vi "资讯打标签-打印函数.vi"(5 "条码类型":bool, 6 "错误输入（无错误）":errorcluster caption="print error in", 7 "label num":i32, 8 "print path local":bool, 9 "PRINT":refnum<k24>, 10 "SN":refnum<k24>, 11 "SN输入":string="000019120-SD-R/Z00A2R1553S") -> (3 "printPath":string, 4 "print error":errorcluster caption="print error out")   [LabVIEW 2011]
uses:
  D:/gitProjects/HPTS_VNA/Data/ClassLibraryMisWebservice.dll
  Data/ClassLibraryMisWebservice.dll
  subVI/logrecord/logrecordstring.vi
panel:
  out "Temp":string
  out "strPrintContent":string
  out "PrintSFCFSNLabel":string="OK"
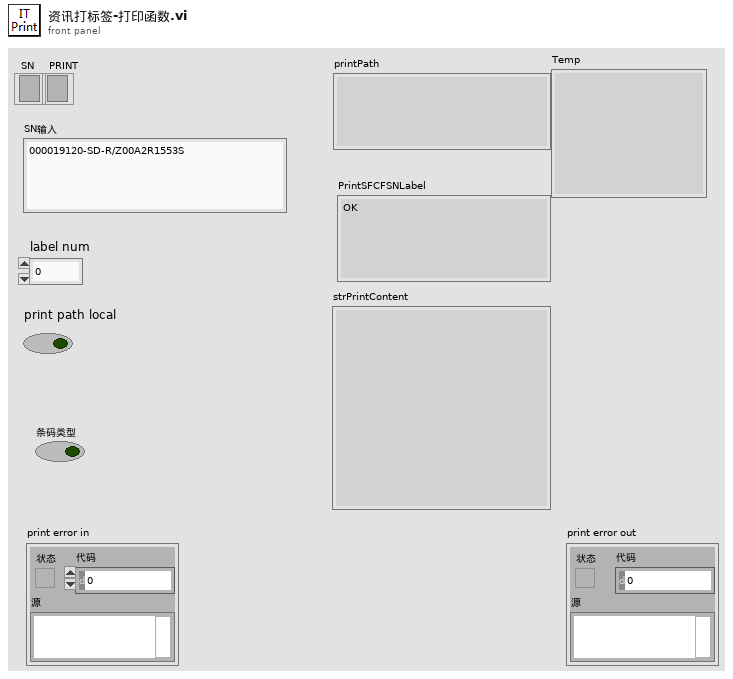
[diagram p1: front panel]
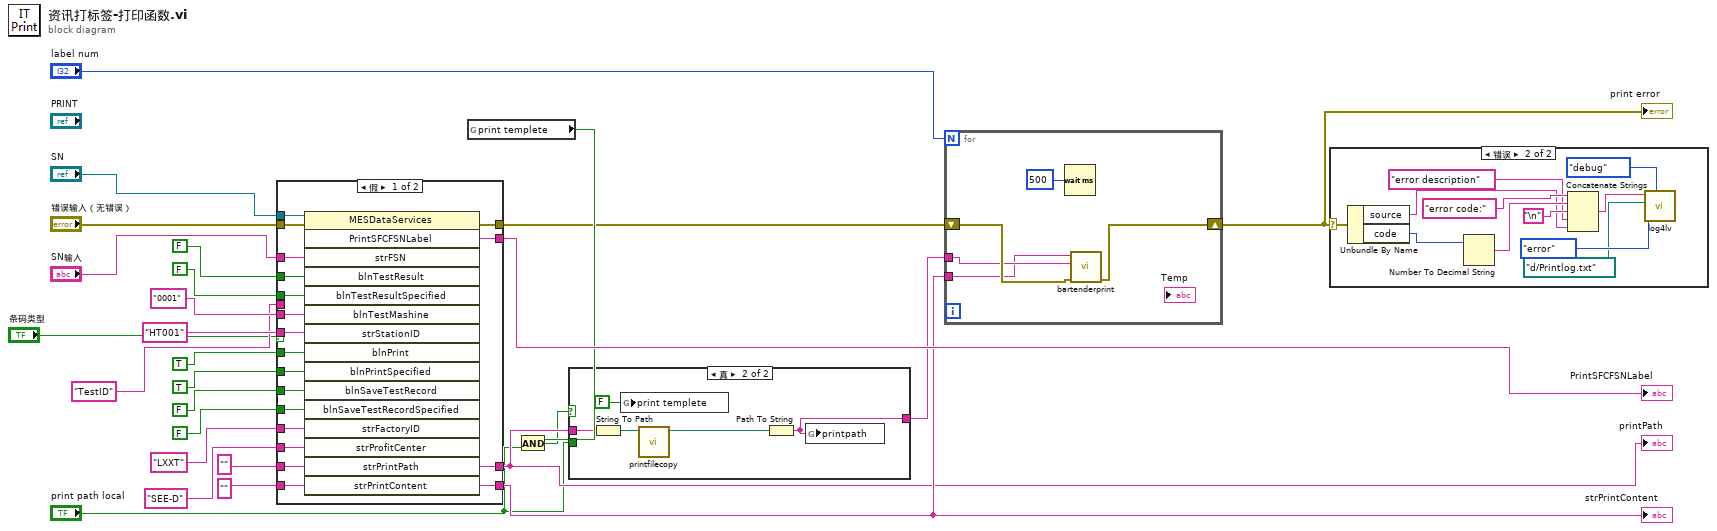
[diagram p0: block diagram]
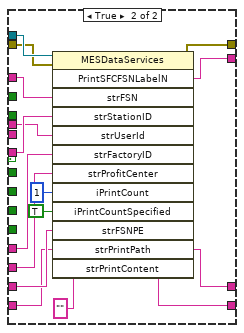
[diagram p2: hidden frame]
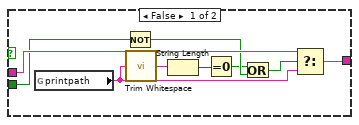
[diagram p4: hidden frame]
diagram:
  n1 = case shown="假" "条码类型" {
    tunnel: FALSE ("blnTestResult") -> [w46 _]
    tunnel: FALSE ("blnTestResultSpecified") -> [w45 _]
    tunnel: "0001" ("blnTestMashine") -> [w44 _]
    tunnel: "HT001" ("strStationID") -> [w43 w57]
    tunnel: TRUE ("blnPrint") -> [w42 _]
    tunnel: TRUE ("blnPrintSpecified") -> [w41 _]
    tunnel: FALSE ("blnSaveTestRecord") -> [w40 _]
    tunnel: FALSE ("blnSaveTestRecordSpecified") -> [w39 _]
    tunnel: "LXXT" ("strFactoryID") -> [w38 w55]
    tunnel: "SEE-D" ("strProfitCenter") -> [w37 w54]
    tunnel: "" ("printPath") -> [w36 w51]
    tunnel: [w35 w58] -> w16
    tunnel: "SN输入" -> [w34 w59]
    tunnel: "" ("strPrintContent") -> [w33 w50]
    tunnel: [w32 w47] -> w13
    tunnel: "SN" -> [w31 w62]
    tunnel: [w30 w48] -> w11
    tunnel: [w29 w60] -> w5
    tunnel: "错误输入（无错误）" -> [w28 w61]
    tunnel: "TestID" -> [_ w56]
    frame False {
      n2 = invoke class="MESDataServices" method="PrintSFCFSNLabel"(reference=w31, error in=w28, "strFSN"=w34, "blnTestResult"=w46, "blnTestResultSpecified"=w45, "blnTestMashine"=w44, "strStationID"=w43, "blnPrint"=w42, "blnPrintSpecified"=w41, "blnSaveTestRecord"=w40, "blnSaveTestRecordSpecified"=w39, "strFactoryID"=w38, "strProfitCenter"=w37, "strPrintPath"=w36, "strPrintContent"=w33) -> (error out=w29:errorcluster, "PrintSFCFSNLabel"=w35:string, "strPrintPath"=w30:string, "strPrintContent"=w32:string)  [unwired: 1 in, 12 out]
    }
    frame True {
      n3 = invoke class="MESDataServices" method="PrintSFCFSNLabelN"(reference=w62, error in=w61, "strFSN"=w59, "strStationID"=w57, "strUserId"=w56, "strFactoryID"=w55, "strProfitCenter"=w54, "iPrintCount"=1, "iPrintCountSpecified"=TRUE, "strFSNPE"=w51, "strPrintPath"=w50, "strPrintContent"="") -> (error out=w60:errorcluster, "PrintSFCFSNLabelN"=w58:string, "strPrintPath"=w48:string, "strPrintContent"=w47:string)  [unwired: 1 in, 9 out]
    }
  }
  "printPath" <- w11
  "PrintSFCFSNLabel" <- w16
  "strPrintContent" <- w13
  n4 = global read "全局.vi" "print templete"() -> (w9:bool)
  n5 = And(x=w9, y="print path local") -> (x .and. y?=w8:bool)
  n6 = case shown="真" w8 {
    tunnel: w11 -> [w69 w76]
    tunnel: [w67 w72] -> w10
    tunnel: "print path local" -> [w66 _]
    frame False {
      n7 = global read "全局.vi" "printpath"() -> (w68:string)
      n8 = Not(x=w66) -> (.not. x?=w65:bool)
      n9 = call <vilib>:"Trim Whitespace.vi"("string"=w68) -> ("trimmed string"=w71:string)  [unwired: 1 in]
      n10 = String Length(string=w71) -> (length=w70:i32)
      n11 = Equal To 0?(x=w70) -> (x = 0?=w64:bool)
      n12 = Or(x=w64, y=w65) -> (x .or. y?=w63:bool)
      n13 = Select(t=w69, s=w63, f=w68) -> (s? t:f=w67:string)
    }
    frame True {
      n14 = String To Path(string=w76) -> (path=w75:path)
      n15 = global write "全局.vi" "print templete"(FALSE ("print templete")) -> ()
      n16 = call "printfilecopy.vi"("源路径"=w75) -> ("new path"=w74:path)  [unwired: 9 in, 1 out]
      n17 = Path To String(path=w74) -> (string=w72:string)
      n18 = global write "全局.vi" "printpath"(w72) -> ()
    }
  }
  n19 = for {
    N: "label num" -> [_]
    tunnel: w13 -> [w77]
    tunnel: w10 -> [w78]
    shift-right: [w80] -> w3
    shift-left: w5 -> [w79]
    n20 = Wait (ms)(milliseconds to wait=u32 500 ("等待时间（毫秒）")) -> ()  [unwired: 1 out]
    n21 = call "bartenderprint.vi"("错误输入"=w79, "Bartender File Path"=w78, "PrintString"=w77) -> ("错误输出"=w80:errorcluster)  [unwired: 8 in]
  }
  "print error" <- w3
  n22 = case shown="错误" w3 {
    selector: w3 -> [_ w92]
    frame No Error {
    }
    frame Error {
      n23 = Unbundle By Name(w92) -> ("source"=w87:string, "code"=w86:i32)
      n24 = Number To Decimal String(number=w86) -> (decimal integer string=w90:string)  [unwired: 1 in]
      n25 = Concatenate Strings("error code:" ("字符串"), w90, "\n", "error description" ("字符串"), w87) -> (w85:string)
      n26 = call-poly "log4lv.vi"("logsetting"=enum16{"error", "info", "debug"}."debug", "logtype"=enum16{"error", "info", "debug"}."error", "LogPath"=path "d:/Printlog.txt", "Msg"=w85) -> ()  [unwired: 7 in, 1 out]
    }
  }
